vi "subGeneratePackets.vi"(0 "Samples per Symbol":i32, 1 "Packet Pad \n[samples]":i32, 3 "PSK system parameters":T2, 5 "Tx IQ Sampling\nRate [s/sec]":dbl, 7 "Pulse Shaping Filter Parameters":T3, 9 "Packet Repeat":i32, 11 "PN sequence order\nfor Sync Bits":i32, 12 "Packet Parameters":T1, 15 "Message Text":string) -> (4 "Number of Packets":i32, 6 "Packets":cluster{"t0":dbl, "dt":dbl, "Y":cdb[]}[](array[cluster]), 8 "error constant":errorcluster, 10 "Symbol Rate":dbl)   [LabVIEW 2023]
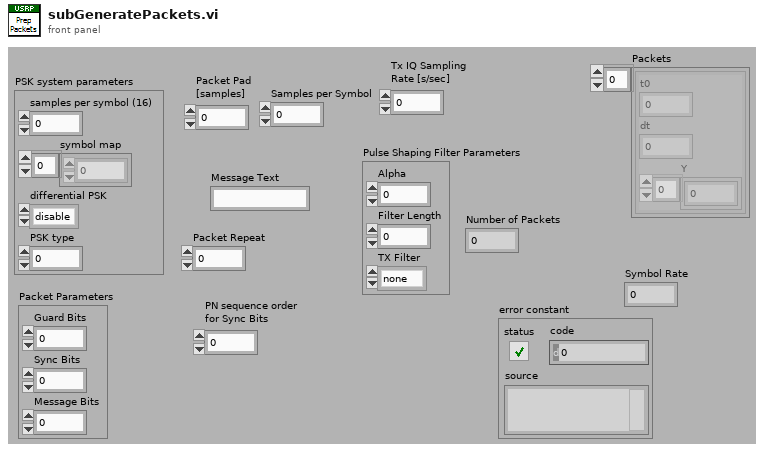
[diagram p1: front panel]
types:
  T1 = cluster{"Guard Bits ":i32, "Sync Bits":i32, "Message Bits":i32}
  T2 = cluster{"samples per symbol (16)":i32, "symbol map":cdb[], "differential PSK":enum16{"disable", "enable"}, "PSK type":u16}
  T3 = cluster{"Alpha":dbl, "Filter Length":i32, "TX Filter":enum16{"none", "Raised Cosine", "Root Raised Cos", "Gaussian"}}
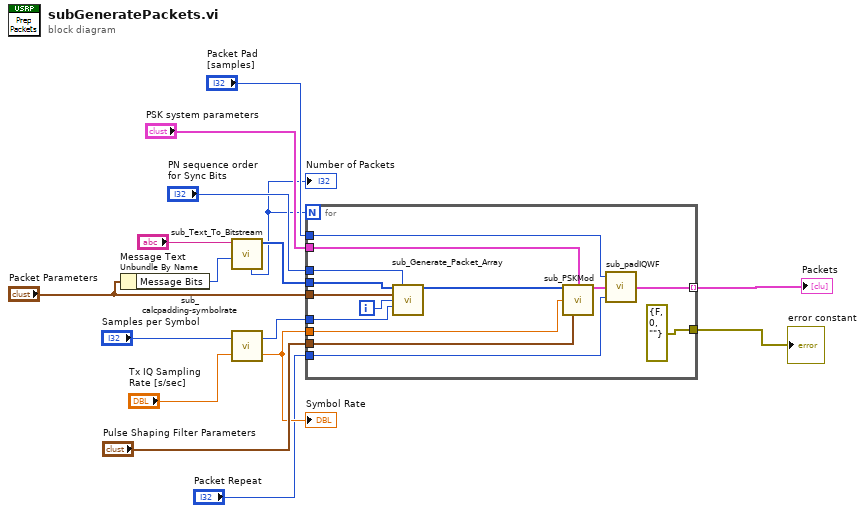
[diagram p0: block diagram]
diagram:
  n1 = Unbundle By Name("Packet Parameters") -> ("Message Bits"=w8:i32)
  n2 = call "sub_Text_To_Bitstream.vi"("Packet\nMessage Length (bits)"=w8, "text"="Message Text") -> ("message bitstream"=w12:i8[], "Number of Packets"=w3:i32)  [unwired: 7 in, 1 out]
  "Number of Packets" <- w3
  n3 = call "sub_calcpadding-symbolrate.vi"("Tx IQ Sampling\nRate [s/sec]"="Tx IQ Sampling\nRate [s/sec]", "Samples per Symbol"="Samples per Symbol") -> ("Symbol Rate"=w5:dbl, "Padding Bits"=w7:i32)
  "Symbol Rate" <- w5
  n4 = for {
    N: w3 -> [_]
    tunnel: "Packet Parameters" -> [w19]
    tunnel: [w24] -> w10 mode=indexing
    tunnel: w12 -> [w21]
    tunnel: "PN sequence order\nfor Sync Bits" -> [w29]
    tunnel: w7 -> [w20]
    tunnel: "PSK system parameters" -> [w27]
    tunnel: w5 -> [w26]
    tunnel: "Pulse Shaping Filter Parameters" -> [w25]
    tunnel: "Packet Pad \n[samples]" -> [w22]
    tunnel: "Packet Repeat" -> [w18]
    tunnel: [errorcluster {"status"=FALSE, "code"=0, "source"=""} ("error constant")] -> w1
    i -> [w30]
    n5 = call "sub_Generate_Packet_Array.vi"("user  bitstream"=w21, "PN sequence order\nfor Sync"=w29, "Packet Parameters"=w19, "Packet Number"=w30, "Cyclic Padding Bits"=w20) -> ("Output Packet"=w28:i8[])  [unwired: 10 in]
    n6 = call "sub_PSKMod.vi"("Packet to Transmit"=w28, "PSK system parameters"=w27, "Symbol Rate, Hz"=w26, "filter parameters"=w25) -> ("output complex waveform"=w23:cluster{"t0":dbl, "dt":dbl, "Y":cdb[]})  [unwired: 10 in, 1 out]
    n7 = call "sub_padIQWF.vi"("Repeat"=w18, "input complex waveform"=w23, "Packet Pad \n[samples]"=w22) -> ("output complex waveform"=w24:cluster{"t0":dbl, "dt":dbl, "Y":cdb[]})
  }
  "Packets" <- w10
  "error constant" <- w1
